vi "Set Reg Domain.vi"(8 "error in (no error)":errorcluster, 10 "regDmn":u32, 11 "_hResourceContext":u32) -> (0 "error out":errorcluster, 2 "regDmn out":u32, 3 "_hResourceContext out":u32)   [LabVIEW 2013, in "QCAWLAN_DLL.lvlib"]
doc: "QCA_DLL_Export void SetRegDomain(HANDLE _hResourceContext, unsigned int *regDmn);"
uses:
  QCAWLAN_DLL.lvlib
  QCAWLAN_DLL.dll
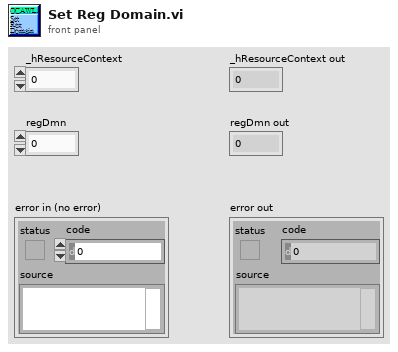
[diagram p1: front panel]
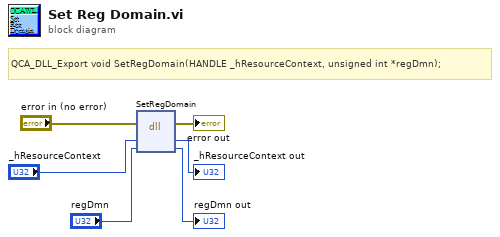
[diagram p0: block diagram]
diagram:
  # "QCA_DLL_Export void SetRegDomain(HANDLE _hResourceContext, unsigned int *regDmn);"
  n1 = dll-call lib="C:/Connectivity Client - MIMO/PlugIn/QCAWLAN_DLL.*" fn="SetRegDomain"(error in="error in (no error)", "_hResourceContext"="_hResourceContext", "regDmn"="regDmn") -> (error out=→"error out":errorcluster, "_hResourceContext"=→"_hResourceContext out":u32, "regDmn"=→"regDmn out":u32)  [unwired: 3 in, 1 out]
